vi "_API Tree.vi"   [LabVIEW 2014]
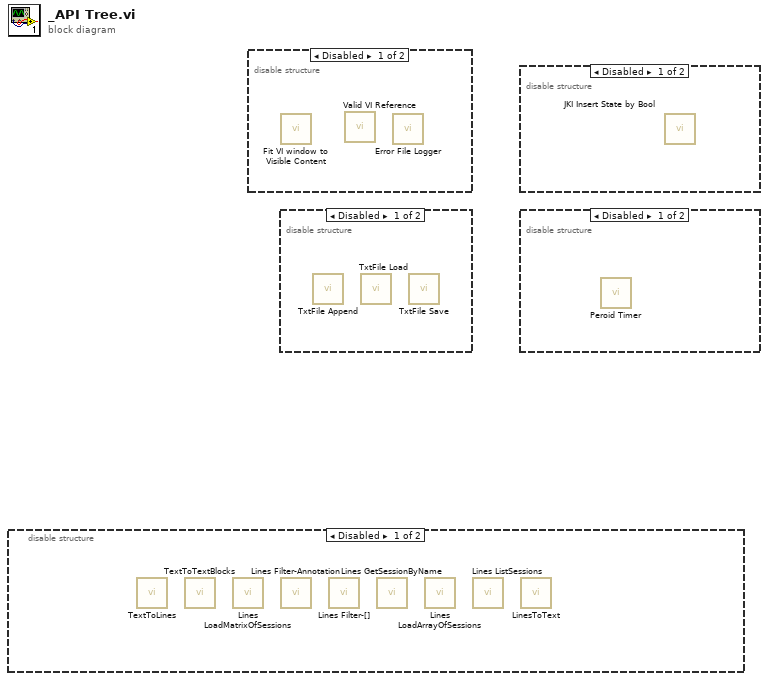
[diagram p0: block diagram]
diagram:
  n1 = disable-structure shown="Disabled" {
    frame Disabled {
      n2 = call "TextToLines.vi"() -> ()  [unwired: 10 in, 2 out]
      n3 = call "TextToTextBlocks.vi"() -> ()  [unwired: 10 in, 2 out]
      n4 = call "Lines LoadMatrixOfSessions.vi"() -> ()  [unwired: 9 in, 3 out]
      n5 = call "Lines Filter-Annotation.vi"() -> ()  [unwired: 10 in, 2 out]
      n6 = call "Lines Filter-[].vi"() -> ()  [unwired: 10 in, 2 out]
      n7 = call "Lines GetSessionByName.vi"() -> ()  [unwired: 9 in, 3 out]
      n8 = call "Lines LoadArrayOfSessions.vi"() -> ()  [unwired: 8 in, 4 out]
      n9 = call "Lines ListSessions.vi"() -> ()  [unwired: 9 in, 3 out]
      n10 = call "LinesToText.vi"() -> ()  [unwired: 10 in, 2 out]
    }
    frame Enabled {
    }
  }
  n11 = disable-structure shown="Disabled" {
    frame Disabled {
      n12 = call "Fit VI window to Visible Content.vi"() -> ()  [unwired: 6 in, 2 out]
      n13 = call "Valid VI Reference.vi"() -> ()  [unwired: 10 in, 1 out]
      n14 = call "Error File Logger.vi"() -> ()  [unwired: 14 in, 2 out]
    }
    frame Enabled {
    }
  }
  n15 = disable-structure shown="Disabled" {
    frame Disabled {
      n16 = call "TxtFile Append.vi"() -> ()  [unwired: 10 in, 2 out]
      n17 = call "TxtFile Load.vi"() -> ()  [unwired: 10 in, 2 out]
      n18 = call "TxtFile Save.vi"() -> ()  [unwired: 11 in, 1 out]
    }
    frame Enabled {
    }
  }
  n19 = disable-structure shown="Disabled" {
    frame Disabled {
      n20 = call "JKI Insert State by Bool.vi"() -> ()  [unwired: 11 in, 1 out]
    }
    frame Enabled {
    }
  }
  n21 = disable-structure shown="Disabled" {
    frame Disabled {
      n22 = call "Peroid Timer.vi"() -> ()  [unwired: 9 in, 2 out]
    }
    frame Enabled {
    }
  }
